vi "FTW-Benchmark-MessageTransports.vi"() -> ()   [LabVIEW 2013]
uses:
  source/actor/Message/Request/FTW-Message-IncomingRequest.lvclass
  source/actor/Ether/FTW-Ether.lvclass
  source/actor/Reply/FTW-Reply.lvclass
  source/actor/Request/FTW-Request.lvclass
panel:
  in  "Client Mode":enum32{"Parallel", "Serial"}(radio)=enum."Serial"
  in  "Number of Clients":i32=8
  out "Results":T1(array[cluster])
  in  "Server Addresses to Test":string[](array[string])=["inproc://*", "tcp://127.0.0.1/*"]
  in  "Requests to Send":i32=500
  in  "stop":bool
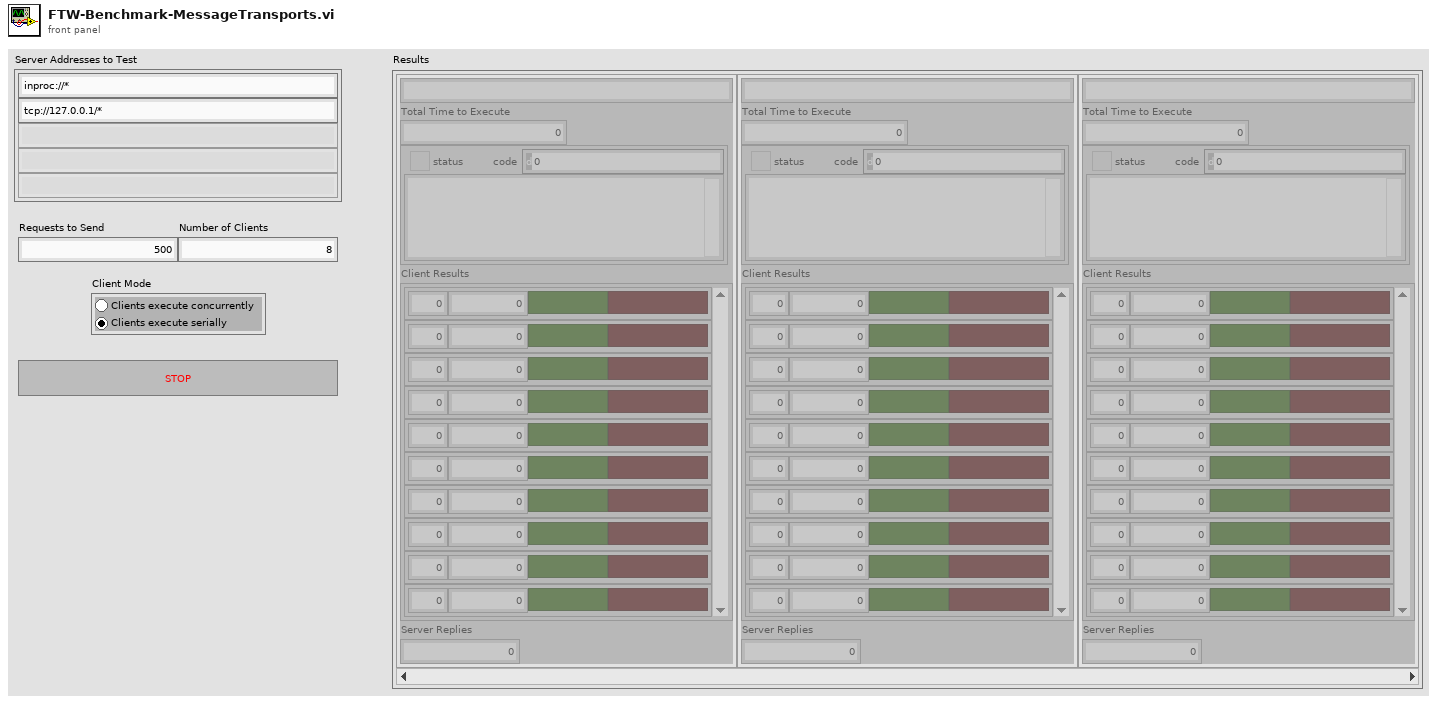
[diagram p1: front panel]
types:
  T1 = cluster{"Server Address":string, "Total Time to Execute":u32, "error":errorcluster, "Client Results":cluster{"Instance":i32, "Requests":i32, "All replies were as expected?":bool, "Timed out?":bool}[], "Server Replies":i32}[]
  T2 = cluster{"Actual Endpoint Address":string, "Elapsed Time":u32, "error out":errorcluster, cluster{i32, i32, bool, bool}[], i32}[]
  T3 = cluster{"Actual Address":string, "Elapsed Time":u32, "error IO":errorcluster, cluster{i32, i32, bool, bool}[], i32}
  T4 = cluster{"Actual Address":string, "Elapsed Time":u32, "error IO":errorcluster, cluster{i32, i32, bool, bool}[], i32}[]
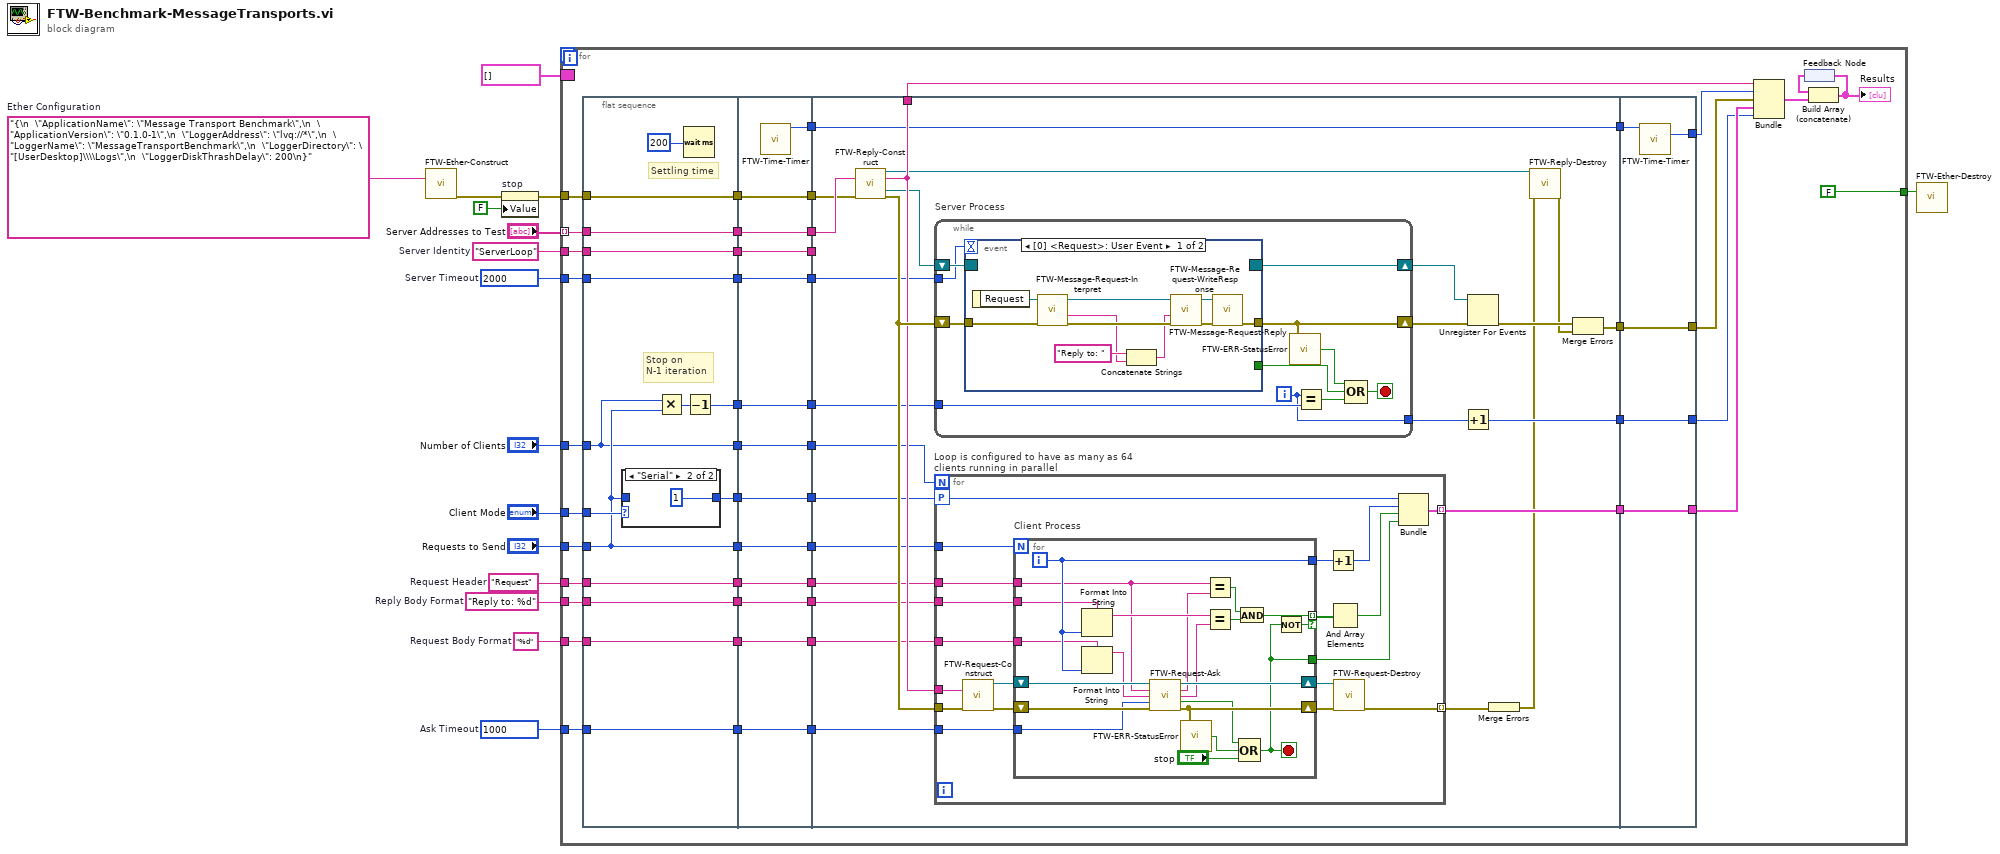
[diagram p0: block diagram]
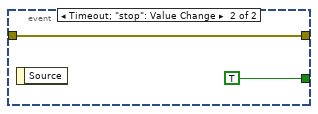
[diagram p3: hidden frame]
diagram:
  w1 = "{\n  \"ApplicationName\": \"Message Transport Benchmark\",\n  \"ApplicationVersion\": \"0.1.0-1\",\n  \"LoggerAddress\": \"lvq://*\",\n  \"LoggerName\": \"MessageTransportBenchmark\",\n  \"LoggerDirectory\": \"[UserDesktop]\\\\Logs\",\n  \"LoggerDiskThrashDelay\": 200\n}"  # Ether Configuration
  w3 = "%d"  # Request Body Format
  w5 = "Request"  # Request Header
  w4 = "Reply to: %d"  # Reply Body Format
  w8 = 1000  # Ask Timeout
  w9 = 2000  # Server Timeout
  w13 = "ServerLoop"  # Server Identity
  n1 = call "FTW-Ether-Construct.vi"("FTW Ether Configuration"=w1) -> ("error out"=w6:errorcluster)  [unwired: 14 in]
  n2 = property on="stop" class="Bool (strict)"(error in=w6, "Value"=FALSE ("stop")) -> (error out=w10:errorcluster)  [unwired: 1 in, 1 out]
  n3 = for {
    tunnel: "Server Addresses to Test" -> [w58] mode=indexing
    tunnel: "Number of Clients" -> [w53]
    tunnel: "Requests to Send" -> [w46]
    tunnel: w13 -> [w42]
    tunnel: "Client Mode" -> [w41]
    tunnel: w10 -> [w40]
    tunnel: w9 -> [w37]
    tunnel: w8 -> [w34]
    border: T2 [] -> [_]
    tunnel: w5 -> [w24]
    tunnel: w4 -> [w21]
    tunnel: w3 -> [w18]
    tunnel: [FALSE ("Force Destroy?")] -> w2
    n4 = flat-sequence {
      tunnel: [w80] -> w65
      tunnel: [w78] -> w59
      tunnel: [w66] -> w54
      tunnel: [w70] -> w47
      tunnel: [w77] -> w43
      tunnel: w40 -> [w80]
      tunnel: w41 -> [w74]
      tunnel: w42 -> [w77]
      tunnel: w46 -> [w70]
      tunnel: w53 -> [w66]
      tunnel: w58 -> [w78]
      tunnel: [w76] -> w38
      tunnel: w37 -> [w76]
      tunnel: [w75] -> w35
      tunnel: w34 -> [w75]
      tunnel: [w73] -> w32
      tunnel: [w71] -> w30
      tunnel: [w69] -> w25
      tunnel: w24 -> [w69]
      tunnel: [w68] -> w22
      tunnel: w21 -> [w68]
      tunnel: [w67] -> w19
      tunnel: w18 -> [w67]
      tunnel: [w95] -> w64
      tunnel: [w94] -> w63
      tunnel: w65 -> [w95]
      tunnel: [w93] -> w60
      tunnel: w59 -> [w93]
      tunnel: [w92] -> w55
      tunnel: w54 -> [w92]
      tunnel: [w91] -> w48
      tunnel: w47 -> [w91]
      tunnel: [w90] -> w44
      tunnel: w43 -> [w90]
      tunnel: [w89] -> w39
      tunnel: w38 -> [w89]
      tunnel: [w88] -> w36
      tunnel: w35 -> [w88]
      tunnel: [w87] -> w33
      tunnel: w32 -> [w87]
      tunnel: [w86] -> w31
      tunnel: w30 -> [w86]
      tunnel: [w85] -> w26
      tunnel: w25 -> [w85]
      tunnel: [w84] -> w23
      tunnel: w22 -> [w84]
      tunnel: [w83] -> w20
      tunnel: w19 -> [w83]
      tunnel: [w99] -> w62
      tunnel: [w117] -> w61
      tunnel: [w116] -> w51
      tunnel: [w115] -> w50
      tunnel: w31 -> [w111]
      tunnel: w33 -> [w102]
      tunnel: w64 -> [w100]
      tunnel: w63 -> [w117]
      tunnel: w60 -> [w101]
      tunnel: w55 -> [w108]
      tunnel: w48 -> [w110]
      tunnel: [w120] -> w45
      tunnel: w44 -> [_]
      tunnel: w39 -> [w107]
      tunnel: w36 -> [w106]
      tunnel: w26 -> [w98]
      tunnel: w23 -> [w97]
      tunnel: w20 -> [w96]
      tunnel: [w189] -> w57
      tunnel: w62 -> [w189]
      tunnel: w61 -> [w188]
      tunnel: [w187] -> w56
      tunnel: [w186] -> w52
      tunnel: w51 -> [w186]
      tunnel: [w185] -> w49
      tunnel: w50 -> [w185]
      frame #0 {
        # "Stop on\nN-1 iteration"
        # "Settling time"
        n5 = case shown="\"Serial\"" w74 {
          tunnel: w70 -> [w81 _]
          tunnel: [w81 1 ("Requests to Send")] -> w73
          frame "Parallel" {
          }
          frame "Serial" {
          }
        }
        n6 = Multiply(x=w66, y=w70) -> (x*y=w72:i32)
        n7 = Wait (ms)(milliseconds to wait=u32 200) -> ()  [unwired: 1 out]
        n8 = Decrement(x=w72) -> (x-1=w71:i32)
      }
      frame #1 {
        n9 = call "FTW-Time-Timer.vi"() -> ("Current Tick Count"=w94:u32)  [unwired: 13 in, 2 out]
      }
      frame #2 {
        n10 = call "FTW-Reply-Construct.vi"("Address"=w101, "error in"=w100) -> ("FTW-Router Out"=w105:refnum<class "FTW-Reply.lvclass">, "Actual Address"=w120:string, "Event Registration Refnum"=w112:refnum<event-registration>, "error out"=w121:errorcluster)  [unwired: 10 in]
        n11 = while "Server Process" {
          shift-right: [w171] -> w113
          shift-left: w112 -> [w172]
          shift-right: [w169] -> w114
          shift-left: w121 -> [w170]
          tunnel: w111 -> [w164]
          tunnel: [w163] -> w109
          tunnel: w107 -> [w162]
          i -> [w163]
          stop <- w165 stop-if-true
          n12 = event shown="[0] <Request>: User Event" {
            selector: w172 -> [_ _]
            dyn-events: [_ _] -> w171
            timeout: w162 -> [_ _]
            tunnel: [_ TRUE] -> w167
            tunnel: w170 -> [w180 w183]
            tunnel: [w181 w183] -> w169
            event User Event {
              n13 = event-data() -> ("Request"=w174:refnum<class "FTW-Message-IncomingRequest.lvclass">)  [unwired: 1 in]
              n14 = call "FTW-Message-Request-Interpret.vi"("error in"=w180, "FTW Incoming Request"=w174) -> ("error out"=w179:errorcluster, "Request Body"=w173:string, "FTW Incoming Request out"=w177:refnum<class "FTW-Message-IncomingRequest.lvclass">)  [unwired: 5 in, 2 out]
              n15 = Concatenate Strings("Reply to: ", w173) -> (w175:string)
              n16 = call "FTW-Message-Request-WriteResponse.vi"("error in"=w179, "Response Body"=w175, "FTW Incoming Request"=w177) -> ("error out"=w178:errorcluster, "FTW Incoming Request out"=w176:refnum<class "FTW-Message-IncomingRequest.lvclass">)  [unwired: 7 in]
              n17 = call "FTW-Message-Request-Reply.vi"("FTW: Reply Error"=w178, "FTW Incoming Request"=w176) -> ("error out"=w181:errorcluster)  [unwired: 8 in, 1 out]
            }
            event Timeout; "stop": Value Change {
              n18 = event-data() -> ()  [unwired: 1 in, 1 out]
            }
          }
          n19 = call "FTW-ERR-StatusError.vi"("error to check"=w169) -> ("Error?"=w168:bool)
          n20 = Equal?(x=w163, y=w164) -> (x = y?=w166:bool)
          n21 = Compound Arithmetic op=OR(w168, w167, w166) -> (w165:bool)
        }
        n22 = for "Loop is configured to have as many as 64 clients running in parallel" {
          N: w108 -> [_]
          tunnel: w121 -> [w124]
          tunnel: w110 -> [w140]
          tunnel: w106 -> [w139]
          workers-P: w102 -> [w133]
          tunnel: [w137] -> w104 mode=indexing
          tunnel: [w136] -> w116 mode=indexing
          tunnel: w120 -> [w122]
          tunnel: w97 -> [w131]
          tunnel: w98 -> [w130]
          tunnel: w96 -> [w129]
          n23 = call "FTW-Request-Construct.vi"("Server Address"=w122, "error in"=w124) -> ("FTW-Request Out"=w125:refnum<class "FTW-Request.lvclass">, "error out"=w123:errorcluster)  [unwired: 12 in]
          n24 = for "Client Process" {
            N: w140 -> [_]
            shift-right: [w159] -> w138
            shift-left: w125 -> [w161]
            tunnel: w139 -> [w155]
            tunnel: [w150] -> w134
            tunnel: [w153] -> w135
            tunnel: [w146] -> w128 mode=indexing if=w141
            tunnel: w131 -> [w152]
            tunnel: w130 -> [w142]
            tunnel: w129 -> [w151]
            shift-right: [w158] -> w126
            shift-left: w123 -> [w160]
            i -> [w153]
            stop <- w150 stop-if-true
            n25 = Format Into String(format string=w152, w153) -> (resulting string=w145:string)  [unwired: 2 in, 1 out]
            n26 = Format Into String(format string=w151, w153) -> (resulting string=w149:string)  [unwired: 2 in, 1 out]
            n27 = call "FTW-Request-Ask.vi"("FTW-Request In"=w161, "Header"=w142, "Body"=w149, "Timeout"=w155, "error in"=w160) -> ("FTW-Request Out"=w159:refnum<class "FTW-Request.lvclass">, "Response Header"=w144:string, "Response Body"=w143:string, "Timed out?"=w154:bool, "error out"=w158:errorcluster)  [unwired: 4 in, 2 out]
            n28 = call "FTW-ERR-StatusError.vi"("error to check"=w158) -> ("Error?"=w157:bool)
            n29 = Equal?(x=w142, y=w144) -> (x = y?=w147:bool)
            n30 = Equal?(x=w145, y=w143) -> (x = y?=w148:bool)
            n31 = And(x=w147, y=w148) -> (x .and. y?=w146:bool)
            n32 = Compound Arithmetic op=OR(w154, w157, "stop") -> (w150:bool)
            n33 = Not(x=w150) -> (.not. x?=w141:bool)
          }
          n34 = Increment(x=w135) -> (x+1=w132:i32)
          n35 = And Array Elements(Boolean array=w128) -> (logical AND=w127:bool)
          n36 = call "FTW-Request-Destroy.vi"("FTW-Request In"=w138, "error in"=w126) -> ("error out"=w137:errorcluster)  [unwired: 13 in]
          n37 = Bundle(w133, w132, w127, w134) -> (w136:cluster{i32, i32, bool, bool})  [unwired: 1 in]
        }
        n38 = Increment(x=w109) -> (x+1=w115:i32)
        n39 = Unregister For Events(event registration refnum=w113, error in=w114) -> (error out=w119:errorcluster)
        n40 = Merge Errors(w104) -> (w103:errorcluster)
        n41 = call "FTW-Reply-Destroy.vi"("FTW-Router In"=w105, "error in"=w103) -> ("error out"=w118:errorcluster)  [unwired: 13 in]
        n42 = Merge Errors(w119, w118) -> (w99:errorcluster)
      }
      frame #3 {
        n43 = call "FTW-Time-Timer.vi"("Initial Tick Count"=w188) -> ("Elapsed Time"=w187:u32)  [unwired: 12 in, 2 out]
      }
    }
    n44 = Bundle("Actual Address"=w45, "Elapsed Time"=w56, "error IO"=w57, w52, w49) -> (w29:T3)  [unwired: 1 in]
    n45 = feedback #1() -> (w28:T2)
    n46 = Build Array (concatenate)(w28, w29) -> (w27:T4)
    "Results" <- w27
    n47 = feedback-in #1(w27) -> ()
  }
  n48 = call "FTW-Ether-Destroy.vi"("Force Destroy?"=w2) -> ()  [unwired: 14 in, 1 out]
